vi "dIMU_Gyro_dps.vi"(7 "Port":T2 items=["Port 1", "Port 2", "Port 3", "Port 4"], 9 "Gyro Scale":u8(ring)=16 items=["250 deg/s"=0, "500 deg/s"=16, "2000 deg/s"=32], 11 "NXT":T1={"Hardware"="NXT", "Flattened String"=""}) -> (0 "Z Gyro (deg/s)":dbl format="%.2f", 1 "Y Gyro (deg/s)":dbl format="%.2f", 2 "X Gyro (deg/s)":dbl format="%.2f", 3 "NXT":T1={"Hardware"="NXT", "Flattened String"=""})   [LabVIEW 2010]
uses:
  <vilib>/NXT/Subs/LVHSConnector.ctl
  <vilib>/NXT/Block Support/NXT_InputPort.ctl
  <vilib>/NXT/Block Support/HWPage.SensorType.ctl
  <vilib>/NXT/Block Support/HWPage.SensorMode.ctl
  <vilib>/NXT/Dual Mode Library/Sensors/i2c_sensors.vi
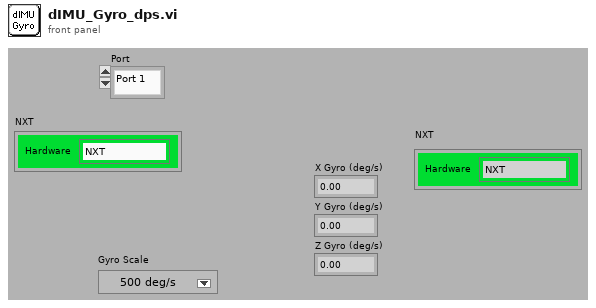
[diagram p1: front panel]
types:
  T1 = typedef "LVHSConnector.ctl" = cluster{"Hardware":string, "Flattened String":string}
  T2 = typedef "NXT_InputPort.ctl" = u8
  T3 = typedef "HWPage.SensorType.ctl" = u8
  T4 = typedef "HWPage.SensorMode.ctl" = u8
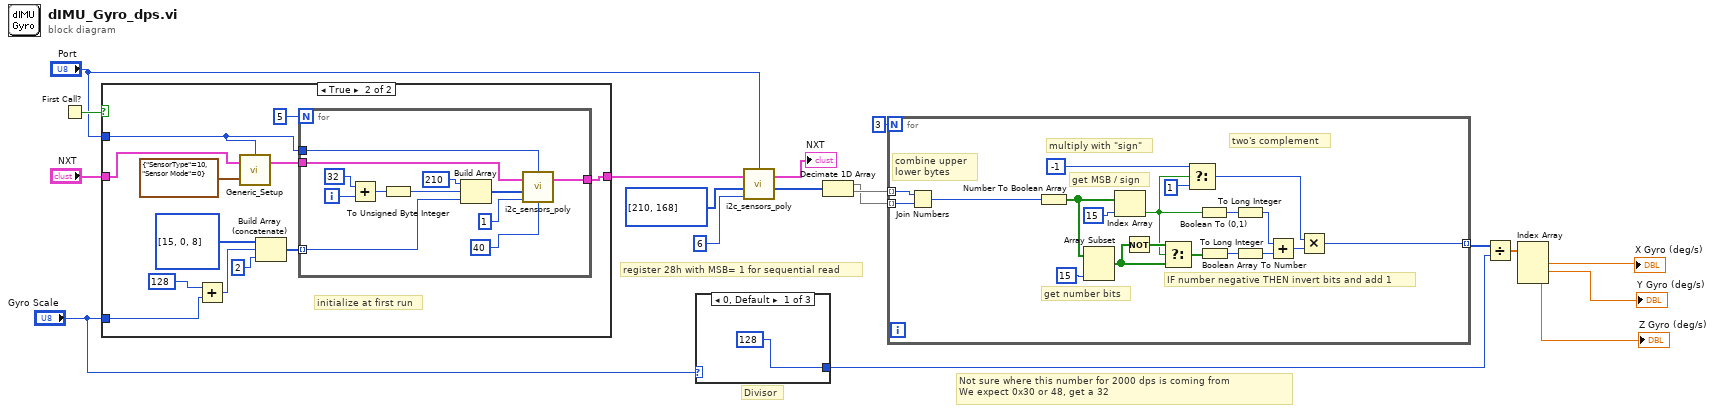
[diagram p0: block diagram]
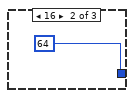
[diagram p2: hidden frame]
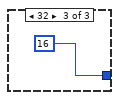
[diagram p3: hidden frame]
diagram:
  # "Not sure where this number for 2000 dps is coming from\nWe expect 0x30 or 48, get a 32"
  # "Divisor"
  # "register 28h with MSB= 1 for sequential read"
  n1 = First Call?() -> (First Call?: T/F=w18:bool)
  n2 = case shown="True" w18 {
    tunnel: [w19 w28] -> w14
    tunnel: "NXT" -> [w19 w27]
    tunnel: "Port" -> [_ w26]
    tunnel: "Gyro Scale" -> [_ w20]
    frame False {
    }
    frame True {
      # "initialize at first run"
      n3 = Add(x=u8 128, y=w20) -> (x+y=w22:u8)
      n4 = call <vilib>:"Generic_Setup.vi"("Sensor Setup"=cluster{"SensorType":T3, "Sensor Mode":T4} {"SensorType"=10, "Sensor Mode"=0}, "NXT"=w27, "Port"=w26) -> ("NXT"=w29:T1)  [unwired: 1 out]
      n5 = Build Array (concatenate)(u8[] [15, 0, 8], w22, u8 2 ("element")) -> (w24:u8[])
      n6 = for {
        N: 5 -> [_]
        tunnel: w29 -> [w43]
        tunnel: w26 -> [w42]
        tunnel: [w33] -> w28
        tunnel: w24 -> [w32] mode=indexing
        i -> [w40]
        n7 = Add(x=32, y=w40) -> (x+y=w38:i32)
        n8 = To Unsigned Byte Integer(number=w38) -> (unsigned 8bit integer=w37:u8)
        n9 = Build Array(u8 210, w37, w32) -> (w36:u8[])
        n10 = call-poly <vilib>:"i2c_sensors_poly.vi"("Return Length"=u8 1, "Bytes to Write"=w36, "Wait (msec)"=u32 40, "NXT"=w43, "Port"=w42) -> ("NXT"=w33:T1)  [unwired: 2 out]
      }
    }
  }
  n11 = case shown="0, Default" "Gyro Scale" {
    tunnel: [u8 128 ("f") u8 64 ("f") u8 16 ("f")] -> w4
    frame 0, Default {
    }
    frame 16 {
    }
    frame 32 {
    }
  }
  n12 = call-poly <vilib>:"i2c_sensors_poly.vi"("Return Length"=u8 6, "Bytes to Write"=u8[] [210, 168], "NXT"=w14, "Port"="Port") -> ("Bytes read"=w8:u8[], "NXT"=→"NXT":T1)  [unwired: 1 in, 1 out]
  n13 = Decimate 1D Array(w8) -> (w11:u8[], w12:u8[])
  n14 = for {
    N: 3 -> [_]
    tunnel: w12 -> [w65] mode=indexing
    tunnel: w11 -> [w64] mode=indexing
    tunnel: [w47] -> w5 mode=indexing
    # "two's complement"
    # "combine upper\nlower bytes"
    # "multiply with \"sign\""
    # "IF number negative THEN invert bits and add 1"
    # "get number bits"
    # "get MSB / sign"
    n15 = Join Numbers(hi=w65, lo=w64) -> ((hi.lo)=w48:u16)
    n16 = Number To Boolean Array(number=w48) -> (Boolean array=w49:bool[])
    n17 = Array Subset(array=w49, length=15) -> (w51:bool[])  [unwired: 1 in]
    n18 = Index Array(array=w49, index=15) -> (element=w52:bool)
    n19 = Not(x=w51) -> (.not. x?=w60:bool[])
    n20 = Select(t=w60, s=w52, f=w51) -> (s? t:f=w50:bool[])
    n21 = Select(t=-1, s=w52, f=1) -> (s? t:f=w55:i32)
    n22 = Boolean To (0,1)(Boolean=w52) -> (0, 1=w58:i16)
    n23 = Boolean Array To Number(Boolean array=w50) -> (number=w61:u32)
    n24 = To Long Integer(number=w58) -> (32bit integer=w53:i32)
    n25 = To Long Integer(number=w61) -> (32bit integer=w59:i32)
    n26 = Add(x=w53, y=w59) -> (x+y=w54:i32)
    n27 = Multiply(x=w55, y=w54) -> (x*y=w47:i32)
  }
  n28 = Divide(x=w5, y=w4) -> (x/y=w6:dbl[])
  n29 = Index Array(array=w6) -> (element #1=→"X Gyro (deg/s)":dbl, element #2=→"Y Gyro (deg/s)":dbl, element #3=→"Z Gyro (deg/s)":dbl)  [unwired: 3 in]
